vi "Write Drag Over  Event Data.vi"(10 "Drag Over  Event Data":refnum<notifier>, 11 "Handle Drag Over Msg in":refnum<class "Handle Drag Over Msg.lvclass">) -> (3 "Handle Drag Over Msg out":refnum<class "Handle Drag Over Msg.lvclass">)   [LabVIEW 2017, in "Handle Drag Over Msg.lvclass"]
uses:
  <vilib>/gpm_packages/@cs/Test-executive-builder/Source/Test Executive Builder View/Test Executive Builder View Messages/Handle Drag Over Msg/Handle Drag Over Msg.lvclass
  <vilib>/gpm_packages/@cs/Test-executive-builder/Source/Test Executive Builder View/Test Executive Builder View Messages/Handle Drag Over Msg/Handle Drag Over Msg.lvclass/Handle Drag Over Msg.ctl
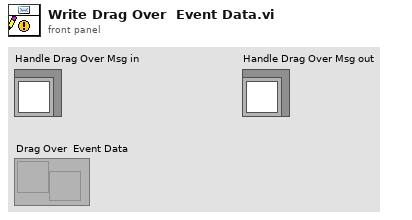
[diagram p1: front panel]
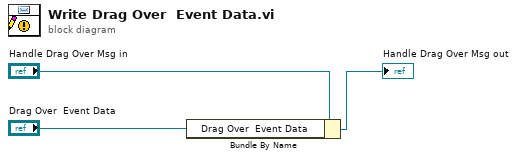
[diagram p0: block diagram]
diagram:
  n1 = Bundle By Name(cluster="Handle Drag Over Msg in", "Drag Over  Event Data"="Drag Over  Event Data") -> (→"Handle Drag Over Msg out":refnum<class "Handle Drag Over Msg.lvclass">)
